vi "Split HDC Bank3 DIO.vi"(0 "IN 7:0":u8) -> (1 "OUT 1:0":fxp<+,2,2>, 2 "OUT 3:2":fxp<+,2,2>, 3 "OUT 5:4":fxp<+,2,2>, 4 "OUT 7:6":fxp<+,2,2>)   [LabVIEW 2015]
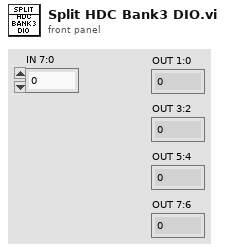
[diagram p1: front panel]
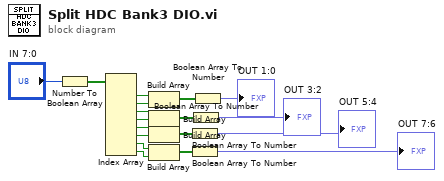
[diagram p0: block diagram]
diagram:
  n1 = Number To Boolean Array(number="IN 7:0") -> (Boolean array=w18:bool[])
  n2 = Index Array(array=w18) -> (element #1=w17:bool, element #2=w16:bool, element #3=w13:bool, element #4=w12:bool, element #5=w10:bool, element #6=w9:bool, element #7=w3:bool, element #8=w2:bool)  [unwired: 8 in]
  n3 = Build Array(w17, w16) -> (w15:bool[])
  n4 = Build Array(w13, w12) -> (w14:bool[])
  n5 = Build Array(w10, w9) -> (w11:bool[])
  n6 = Build Array(w3, w2) -> (w4:bool[])
  n7 = Boolean Array To Number(Boolean array=w11) -> (number=→"OUT 5:4":fxp<+,2,2>)
  n8 = Boolean Array To Number(Boolean array=w4) -> (number=→"OUT 7:6":fxp<+,2,2>)
  n9 = Boolean Array To Number(Boolean array=w14) -> (number=→"OUT 3:2":fxp<+,2,2>)
  n10 = Boolean Array To Number(Boolean array=w15) -> (number=→"OUT 1:0":fxp<+,2,2>)
